vi "Update Previous Button Visibility.vi"(8 "error in (no error)":errorcluster, 11 "Test Channel Model in":refnum<class "Test Channel Model.lvclass">) -> (0 "error out":errorcluster, 3 "Test Channel Model out":refnum<class "Test Channel Model.lvclass">)   [LabVIEW 2013, in "Test Channel Model.lvlib" / "Test Channel Model.lvclass"]
uses:
  Test Channel Model.lvclass
  Test Channel Model.lvclass/Test Channel Model.ctl
  <vilib>/ActorFrameworkMVC/View Observer/View Registry/View Registry.lvclass/View Registry.ctl
  Test Channel Model Messages/Abstract Test Channel Previous Button Visibility Msg/Abstract Test Channel Previous Button Visibility Msg.lvclass
  <vilib>/ActorFrameworkMVC/View Observer/Data Message/Data Message.lvclass
  <vilib>/ActorFrameworkMVC/View Observer/View Registry/View Registry.lvclass
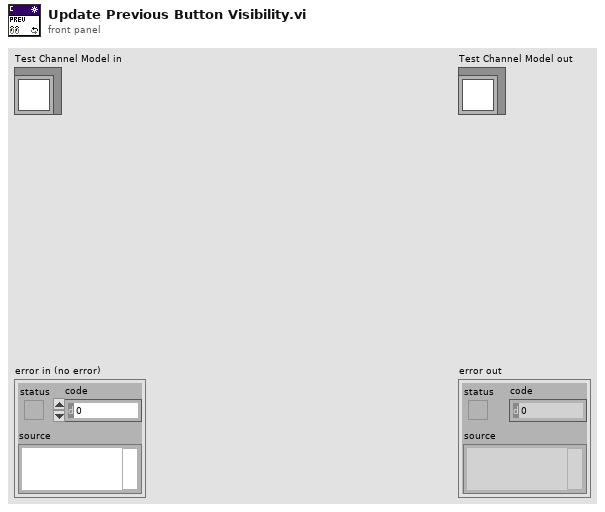
[diagram p1: front panel]
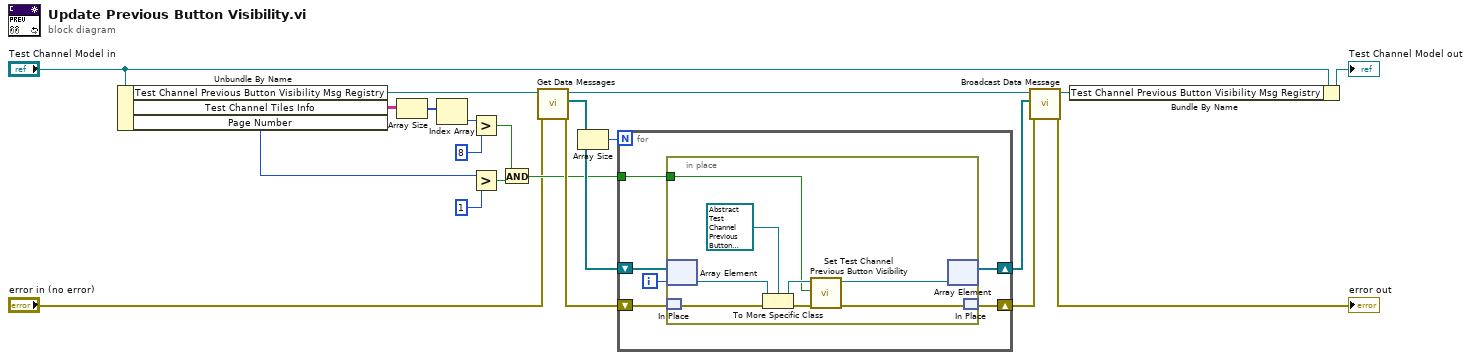
[diagram p0: block diagram]
diagram:
  n1 = Unbundle By Name("Test Channel Model in") -> ("Test Channel Previous Button Visibility Msg Registry"=w21:refnum<class "View Registry.lvclass">, "Test Channel Tiles Info"=w7:string[][], "Page Number"=w6:i32)
  n2 = Array Size(array=w7) -> (size(s)=w12:i32[])
  n3 = Index Array(array=w12) -> (element=w9:i32)  [unwired: 1 in]
  n4 = Greater?(x=w9, y=8) -> (0:w11:bool)
  n5 = Greater?(x=w6, y=1) -> (0:w13:bool)
  n6 = And(x=w11, y=w13) -> (x .and. y?=w5:bool)
  n7 = call <vilib>:"Get Data Messages.vi"("error in (no error)"="error in (no error)", "View Registry in"=w21) -> ("error out"=w17:errorcluster, "Data Messages"=w18:refnum<class "Data Message.lvclass">[], "View Registry out"=w20:refnum<class "View Registry.lvclass">)  [unwired: 7 in]
  n8 = Array Size(array=w18) -> (size(s)=w19:i32)
  n9 = for {
    N: w19 -> [_]
    shift-right: [w26] -> w16
    shift-left: w18 -> [w27]
    shift-right: [w24] -> w15
    shift-left: w17 -> [w25]
    tunnel: w5 -> [w22]
    i -> [w23]
    n10 = in-place {
      in-place-border: w22 -> [w28]
      n11 = in-place-array #1(w27, w23) -> (w33:refnum<class "Data Message.lvclass">)
      n12 = in-place-match #2(w25) -> (w35:errorcluster)
      n13 = To More Specific Class(target class=refnum<class "Abstract Test Channel Previous Button Visibility Msg.lvclass"> refnum ("Test Channel Model.lvlib:Abstract Test Channel Previous Button Visibility Msg.lvclass"), reference=w33, error in=w35) -> (specific class reference=w29:refnum<class "Abstract Test Channel Previous Button Visibility Msg.lvclass">, error out=w32:errorcluster)
      n14 = call "Set Test Channel Previous Button Visibility.vi"("error in (no error)"=w32, "Test Channel Previous Button Visibility"=w28, "Abstract Test Channel Previous Button Visibility Msg in"=w29) -> ("error out"=w31:errorcluster, "Abstract Test Channel Previous Button Visibility Msg out"=w30:refnum<class "Abstract Test Channel Previous Button Visibility Msg.lvclass">)  [unwired: 7 in]
      n15 = in-place-array #1(w30) -> (w26:refnum<class "Data Message.lvclass">[])  [unwired: 1 out]
      n16 = in-place-match #2(w31) -> (w24:errorcluster)
    }
  }
  n17 = call <vilib>:"Broadcast Data Message.vi"("error in (no error)"=w15, "Data Messages"=w16, "View Registry in"=w20) -> ("error out"=→"error out":errorcluster, "View Registry out"=w14:refnum<class "View Registry.lvclass">)  [unwired: 7 in]
  n18 = Bundle By Name(cluster="Test Channel Model in", "Test Channel Previous Button Visibility Msg Registry"=w14) -> (→"Test Channel Model out":refnum<class "Test Channel Model.lvclass">)
